vi "configure_new_target.vi"(11 "vsd":refnum<k24>) -> ()   [LabVIEW 2020]
uses:
  controls/target_configuration_cluster.ctl
  controls/thread_configuration_data.ctl
  controls/tx_transfer_group_configuration_data.ctl
  <vilib>/addons/VeriStand Custom Device Scripting APIs/Data Sharing Framework/DSF Core.lvlibp/Typedefs/DSF Timing Info.ctl
  controls/tx_configuration_data.ctl
  controls/rx_transfer_group_configuration_data.ctl
  controls/rx_configuration_data.ctl
  NationalInstruments.VeriStand.SystemDefinitionAPI
  <vilib>/addons/VeriStand Custom Device Scripting APIs/Data Sharing Framework/DSF Core.lvlibp
panel:
  in  "Remove RX Transfer Group":bool
  in  "Remove RX Connection":bool
  in  "Clear Configuration":bool
  in  "Remove Thread":bool
  in  "Remove TX Transfer Group":bool
  in  "Remove TX Connection":bool
  in  "Finish":bool
  in  "Cancel":bool
  in  "Target Plugin Timing":T1={"priority"=10000, "decimation"=0, "offset"=0}
  in  "Target DSF Threads":T2[](array[typedef])
  in  "Target ID":T7={"Name"="", "IP"="", "Username"="", "Password"="", "Operating System"="Linux_x64"}
  # "Target Settings"
  # "DSF Configuration"
  # "* Decimation = 0 forces \nplugin to be inline with PCL"
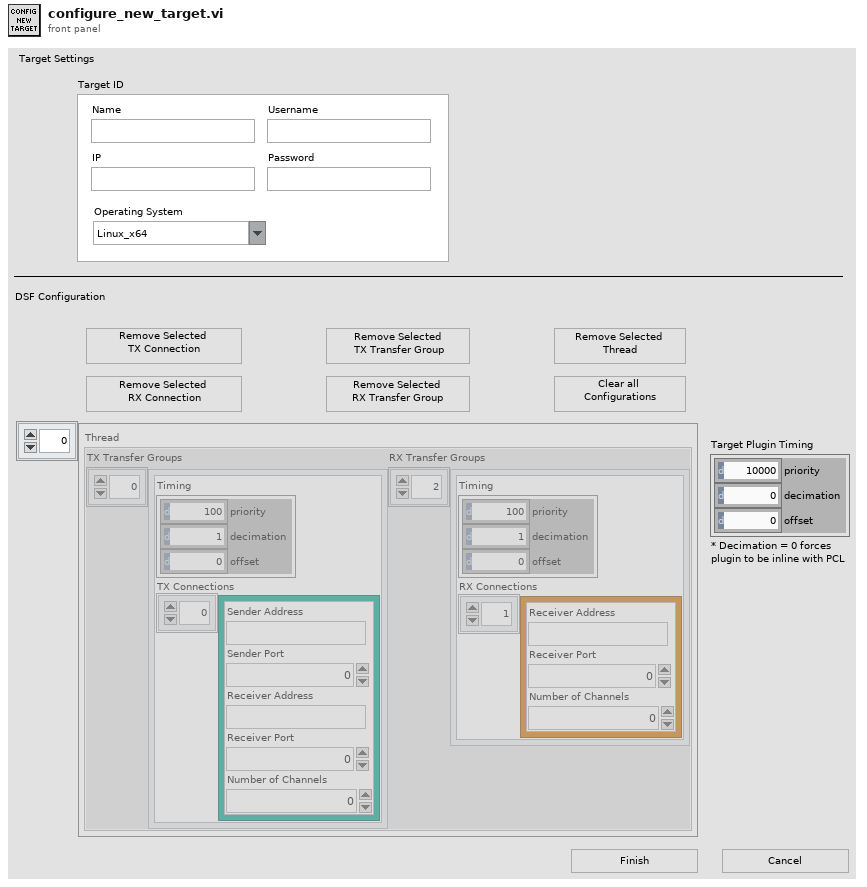
[diagram p1: front panel]
types:
  T1 = typedef "DSF Core.lvlibp/DSF Timing Info.ctl" = cluster{"priority":u64, "decimation":u64, "offset":u64}
  T2 = typedef "thread_configuration_data.ctl" = cluster{"TX Transfer Groups":T3[], "RX Transfer Groups":T5[]}
  T3 = typedef "tx_transfer_group_configuration_data.ctl" = cluster{"Timing":T1, "TX Connections":T4[]}
  T4 = typedef "tx_configuration_data.ctl" = cluster{"Sender Address":string, "Sender Port":u16, "Receiver Address":string, "Receiver Port":u16, "Number of Channels":u16}
  T5 = typedef "rx_transfer_group_configuration_data.ctl" = cluster{"Timing":T1, "RX Connections":T6[]}
  T6 = typedef "rx_configuration_data.ctl" = cluster{"Receiver Address":string, "Receiver Port":u16, "Number of Channels":u16}
  T7 = typedef "target_configuration_cluster.ctl" = cluster{"Name":string, "IP":string, "Username":string, "Password":string, "Operating System":string}
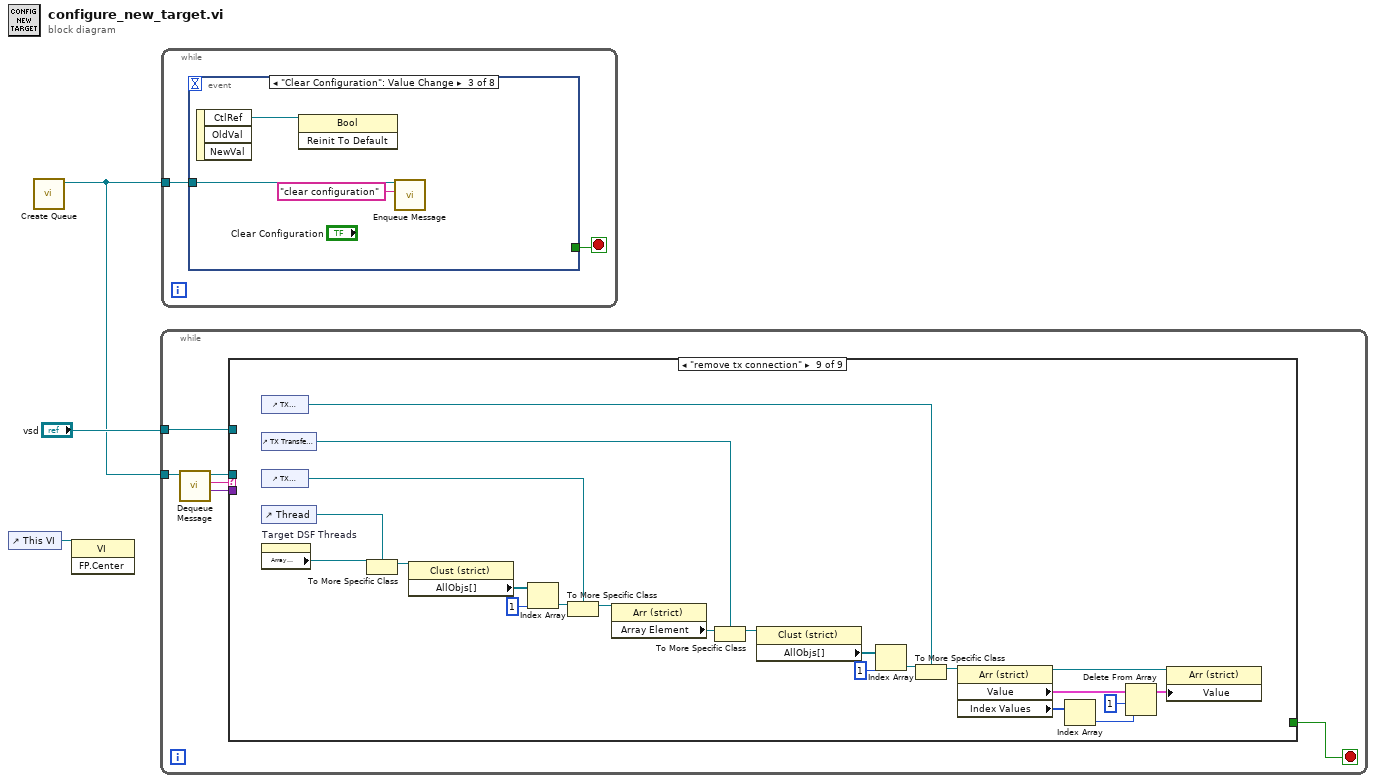
[diagram p0: block diagram]
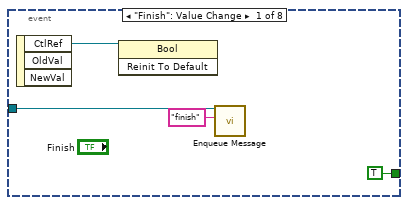
[diagram p2: hidden frame]
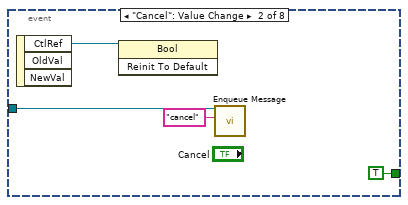
[diagram p3: hidden frame]
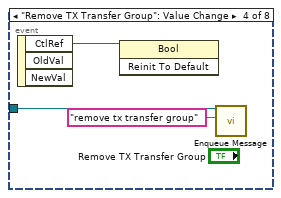
[diagram p4: hidden frame]
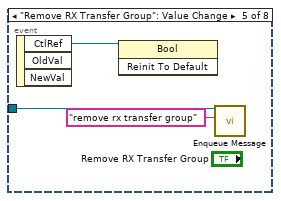
[diagram p5: hidden frame]
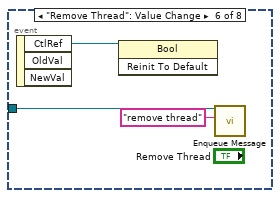
[diagram p6: hidden frame]
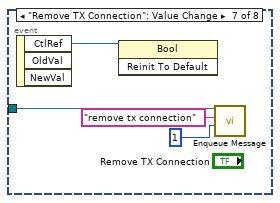
[diagram p7: hidden frame]
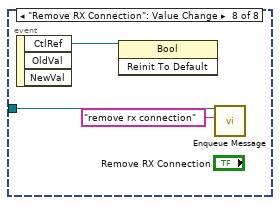
[diagram p8: hidden frame]
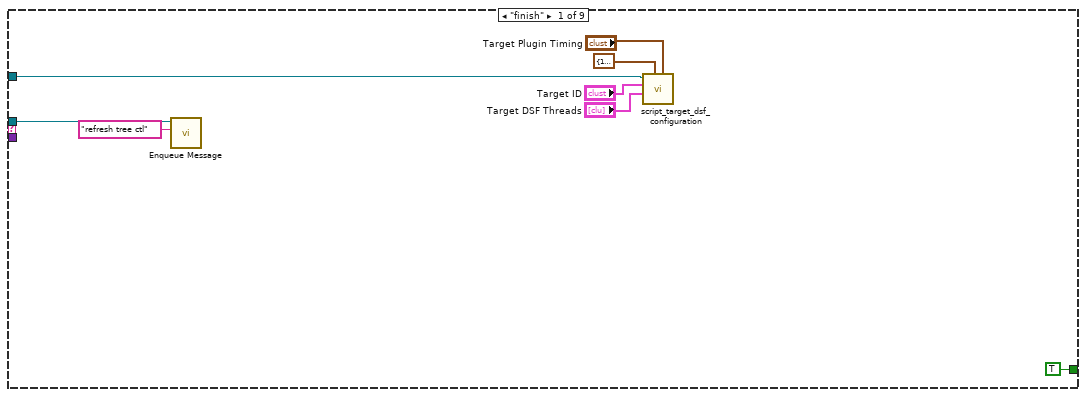
[diagram p9: hidden frame]
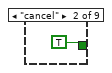
[diagram p10: hidden frame]
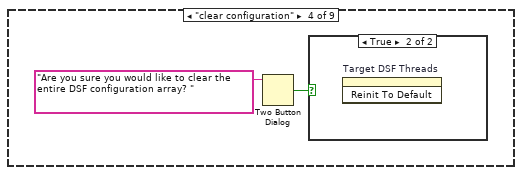
[diagram p12: hidden frame]
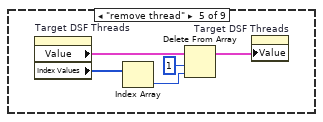
[diagram p14: hidden frame]
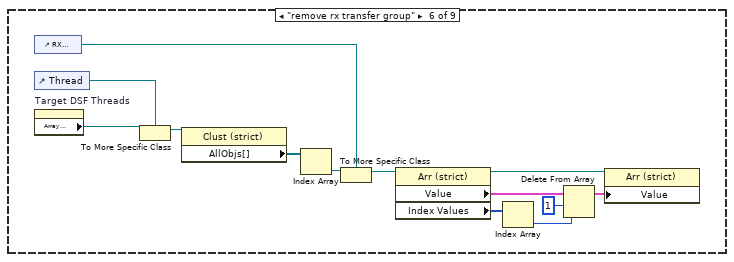
[diagram p15: hidden frame]
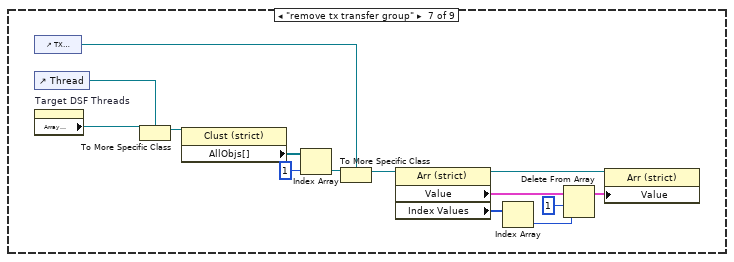
[diagram p16: hidden frame]
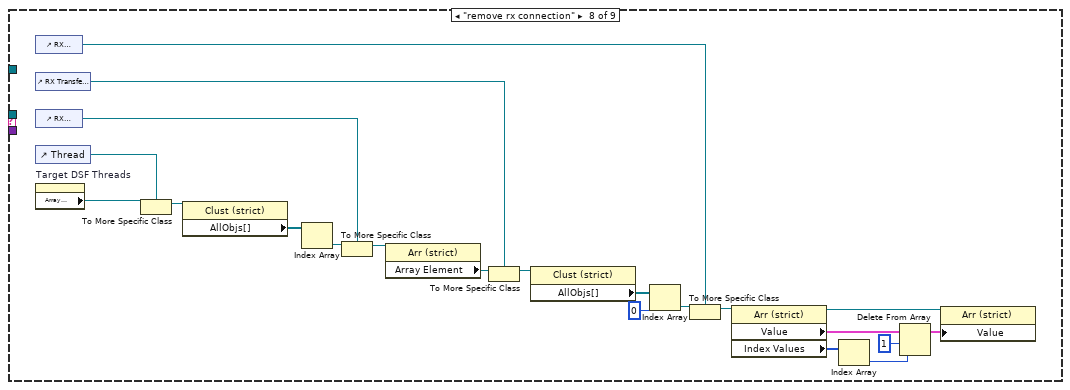
[diagram p17: hidden frame]
diagram:
  n1 = control-ref of="This VI"() -> (w1:refnum<vi>)
  n2 = call "Create Queue.vi"() -> ("Message Queue Out"=w2:refnum<queue>)  [unwired: 10 in, 1 out]
  n3 = invoke class="VI" method="FP.Center"(reference=w1) -> ()  [unwired: 2 in, 3 out]
  n4 = while {
    tunnel: w2 -> [w8]
    tunnel: "vsd" -> [w5]
    stop <- w4 stop-if-true
    n5 = call "Dequeue Message.vi"("Message Queue"=w8) -> ("Message Data"=w6:variant, "Message"=w9:string, "dup Message Queue"=w7:refnum<queue>)  [unwired: 7 in, 1 out]
    n6 = case shown="\"remove tx connection\"" w9 {
      tunnel: w7 -> [w16 _ _ _ _ _ _ _ _]
      tunnel: w6 -> [_ _ _ _ _ _ _ _ _]
      tunnel: w5 -> [w12 _ _ _ _ _ _ _ _]
      tunnel: [TRUE TRUE _ _ _ _ _ _ _] -> w4
      frame "finish" {
        n7 = call "Enqueue Message.vi"("Message"="refresh tree ctl", "Message Queue"=w16) -> ()  [unwired: 8 in, 2 out]
        n8 = call "script_target_dsf_configuration.vi"("Plugin Timing"="Target Plugin Timing", "configuration version"=cluster{"major":u32, "minor":u32, "fix":u32} {"major"=1, "minor"=0, "fix"=0}, "Target Threads"="Target DSF Threads", "Target Configuration"="Target ID", "vsd reference"=w12) -> ()  [unwired: 6 in, 1 out]
      }
      frame "cancel" {
      }
      frame Default {
      }
      frame "clear configuration" {
        n9 = Two Button Dialog(message="Are you sure you would like to clear the entire DSF configuration array? ") -> (T button?=w19:bool)  [unwired: 2 in]
        n10 = case shown="True" w19 {
          frame False {
          }
          frame True {
            n11 = invoke on="Target DSF Threads" class="Arr (strict)" method="Reinit To Default"() -> ()  [unwired: 3 in, 3 out]
          }
        }
      }
      frame "remove thread" {
        n12 = property on="Target DSF Threads" class="Arr (strict)"() -> ("Value"=w24:T2[], "Index Values"=w25:u32[])  [unwired: 2 in, 2 out]
        n13 = Index Array(array=w25) -> (element=w22:u32)  [unwired: 1 in]
        n14 = Delete From Array(array=w24, length=1, index=w22) -> (array with subset deleted=w21:T2[])  [unwired: 1 out]
        n15 = property on="Target DSF Threads" class="Arr (strict)"("Value"=w21) -> ()  [unwired: 2 in, 2 out]
      }
      frame "remove rx transfer group" {
        n16 = control-ref of="RX Transfer Groups"() -> (w27:refnum<vi>)
        n17 = control-ref of="Thread"() -> (w34:refnum<vi>)
        n18 = property on="Target DSF Threads" class="Arr (strict)"() -> ("Array Element"=w38:refnum<vi>)  [unwired: 2 in, 2 out]
        n19 = To More Specific Class(target class=w34, reference=w38) -> (specific class reference=w37:refnum<vi>)  [unwired: 1 in, 1 out]
        n20 = property class="Clust (strict)"(reference=w37) -> ("AllObjs[]"=w36:refnum<vi>[])  [unwired: 1 in, 2 out]
        n21 = Index Array(array=w36) -> (element=w35:refnum<vi>)  [unwired: 1 in]
        n22 = To More Specific Class(target class=w27, reference=w35) -> (specific class reference=w26:refnum<vi>)  [unwired: 1 in, 1 out]
        n23 = property class="Arr (strict)"(reference=w26) -> (reference out=w33:refnum<vi>, "Value"=w29:T5[], "Index Values"=w31:u32[])  [unwired: 1 in, 1 out]
        n24 = Index Array(array=w31) -> (element=w30:u32)  [unwired: 1 in]
        n25 = Delete From Array(array=w29, length=1, index=w30) -> (array with subset deleted=w28:T5[])  [unwired: 1 out]
        n26 = property class="Arr (strict)"(reference=w33, "Value"=w28) -> ()  [unwired: 1 in, 2 out]
      }
      frame "remove tx transfer group" {
        n27 = control-ref of="TX Transfer Groups"() -> (w41:refnum<vi>)
        n28 = control-ref of="Thread"() -> (w48:refnum<vi>)
        n29 = property on="Target DSF Threads" class="Arr (strict)"() -> ("Array Element"=w52:refnum<vi>)  [unwired: 2 in, 2 out]
        n30 = To More Specific Class(target class=w48, reference=w52) -> (specific class reference=w51:refnum<vi>)  [unwired: 1 in, 1 out]
        n31 = property class="Clust (strict)"(reference=w51) -> ("AllObjs[]"=w50:refnum<vi>[])  [unwired: 1 in, 2 out]
        n32 = Index Array(array=w50, index=1) -> (element=w49:refnum<vi>)
        n33 = To More Specific Class(target class=w41, reference=w49) -> (specific class reference=w40:refnum<vi>)  [unwired: 1 in, 1 out]
        n34 = property class="Arr (strict)"(reference=w40) -> (reference out=w47:refnum<vi>, "Value"=w43:T3[], "Index Values"=w45:u32[])  [unwired: 1 in, 1 out]
        n35 = Index Array(array=w45) -> (element=w44:u32)  [unwired: 1 in]
        n36 = Delete From Array(array=w43, length=1, index=w44) -> (array with subset deleted=w42:T3[])  [unwired: 1 out]
        n37 = property class="Arr (strict)"(reference=w47, "Value"=w42) -> ()  [unwired: 1 in, 2 out]
      }
      frame "remove rx connection" {
        n38 = control-ref of="RX Connections"() -> (w64:refnum<vi>)
        n39 = control-ref of="RX Transfer Group"() -> (w68:refnum<vi>)
        n40 = control-ref of="RX Transfer Groups"() -> (w56:refnum<vi>)
        n41 = control-ref of="Thread"() -> (w69:refnum<vi>)
        n42 = property on="Target DSF Threads" class="Arr (strict)"() -> ("Array Element"=w73:refnum<vi>)  [unwired: 2 in, 2 out]
        n43 = To More Specific Class(target class=w69, reference=w73) -> (specific class reference=w72:refnum<vi>)  [unwired: 1 in, 1 out]
        n44 = property class="Clust (strict)"(reference=w72) -> ("AllObjs[]"=w71:refnum<vi>[])  [unwired: 1 in, 2 out]
        n45 = Index Array(array=w71) -> (element=w70:refnum<vi>)  [unwired: 1 in]
        n46 = To More Specific Class(target class=w56, reference=w70) -> (specific class reference=w55:refnum<vi>)  [unwired: 1 in, 1 out]
        n47 = property class="Arr (strict)"(reference=w55) -> ("Array Element"=w54:refnum<vi>)  [unwired: 1 in, 2 out]
        n48 = To More Specific Class(target class=w68, reference=w54) -> (specific class reference=w67:refnum<vi>)  [unwired: 1 in, 1 out]
        n49 = property class="Clust (strict)"(reference=w67) -> ("AllObjs[]"=w65:refnum<vi>[])  [unwired: 1 in, 2 out]
        n50 = Index Array(array=w65, index=0) -> (element=w66:refnum<vi>)
        n51 = To More Specific Class(target class=w64, reference=w66) -> (specific class reference=w61:refnum<vi>)  [unwired: 1 in, 1 out]
        n52 = property class="Arr (strict)"(reference=w61) -> (reference out=w63:refnum<vi>, "Value"=w58:T6[], "Index Values"=w60:u32[])  [unwired: 1 in, 1 out]
        n53 = Index Array(array=w60) -> (element=w59:u32)  [unwired: 1 in]
        n54 = Delete From Array(array=w58, length=1, index=w59) -> (array with subset deleted=w57:T6[])  [unwired: 1 out]
        n55 = property class="Arr (strict)"(reference=w63, "Value"=w57) -> ()  [unwired: 1 in, 2 out]
      }
      frame "remove tx connection" {
        n56 = control-ref of="TX Connections"() -> (w86:refnum<vi>)
        n57 = control-ref of="TX Transfer Group"() -> (w90:refnum<vi>)
        n58 = control-ref of="TX Transfer Groups"() -> (w78:refnum<vi>)
        n59 = control-ref of="Thread"() -> (w91:refnum<vi>)
        n60 = property on="Target DSF Threads" class="Arr (strict)"() -> ("Array Element"=w95:refnum<vi>)  [unwired: 2 in, 2 out]
        n61 = To More Specific Class(target class=w91, reference=w95) -> (specific class reference=w94:refnum<vi>)  [unwired: 1 in, 1 out]
        n62 = property class="Clust (strict)"(reference=w94) -> ("AllObjs[]"=w93:refnum<vi>[])  [unwired: 1 in, 2 out]
        n63 = Index Array(array=w93, index=1) -> (element=w92:refnum<vi>)
        n64 = To More Specific Class(target class=w78, reference=w92) -> (specific class reference=w77:refnum<vi>)  [unwired: 1 in, 1 out]
        n65 = property class="Arr (strict)"(reference=w77) -> ("Array Element"=w76:refnum<vi>)  [unwired: 1 in, 2 out]
        n66 = To More Specific Class(target class=w90, reference=w76) -> (specific class reference=w89:refnum<vi>)  [unwired: 1 in, 1 out]
        n67 = property class="Clust (strict)"(reference=w89) -> ("AllObjs[]"=w87:refnum<vi>[])  [unwired: 1 in, 2 out]
        n68 = Index Array(array=w87, index=1) -> (element=w88:refnum<vi>)
        n69 = To More Specific Class(target class=w86, reference=w88) -> (specific class reference=w83:refnum<vi>)  [unwired: 1 in, 1 out]
        n70 = property class="Arr (strict)"(reference=w83) -> (reference out=w85:refnum<vi>, "Value"=w80:T4[], "Index Values"=w82:u32[])  [unwired: 1 in, 1 out]
        n71 = Index Array(array=w82) -> (element=w81:u32)  [unwired: 1 in]
        n72 = Delete From Array(array=w80, length=1, index=w81) -> (array with subset deleted=w79:T4[])  [unwired: 1 out]
        n73 = property class="Arr (strict)"(reference=w85, "Value"=w79) -> ()  [unwired: 1 in, 2 out]
      }
    }
  }
  n74 = while {
    tunnel: w2 -> [w97]
    stop <- w96 stop-if-true
    n75 = event shown="[2] \"Clear Configuration\": Value Change" {
      selector: _ -> [_ _ _ _ _ _ _ _]
      dyn-events: _ -> [_ _ _ _ _ _ _ _]
      timeout: _ -> [_ _ _ _ _ _ _ _]
      tunnel: w97 -> [w101 w105 w108 w111 w114 w117 w121 w124]
      tunnel: [TRUE TRUE _ _ _ _ _ _] -> w96
      event "Finish": Value Change {
        n76 = event-data() -> ("CtlRef"=w99:refnum<vi>)  [unwired: 1 in, 2 out]
        n77 = invoke class="Bool" method="Reinit To Default"(reference=w99) -> ()  [unwired: 2 in, 3 out]
        n78 = call "Enqueue Message.vi"("Message"="finish", "Message Queue"=w101) -> ()  [unwired: 8 in, 2 out]
      }
      event "Cancel": Value Change {
        n79 = event-data() -> ("CtlRef"=w103:refnum<vi>)  [unwired: 1 in, 2 out]
        n80 = invoke class="Bool" method="Reinit To Default"(reference=w103) -> ()  [unwired: 2 in, 3 out]
        n81 = call "Enqueue Message.vi"("Message"="cancel", "Message Queue"=w105) -> ()  [unwired: 8 in, 2 out]
      }
      event "Clear Configuration": Value Change {
        n82 = event-data() -> ("CtlRef"=w106:refnum<vi>)  [unwired: 1 in, 2 out]
        n83 = invoke class="Bool" method="Reinit To Default"(reference=w106) -> ()  [unwired: 2 in, 3 out]
        n84 = call "Enqueue Message.vi"("Message"="clear configuration", "Message Queue"=w108) -> ()  [unwired: 8 in, 2 out]
      }
      event "Remove TX Transfer Group": Value Change {
        n85 = event-data() -> ("CtlRef"=w109:refnum<vi>)  [unwired: 1 in, 2 out]
        n86 = invoke class="Bool" method="Reinit To Default"(reference=w109) -> ()  [unwired: 2 in, 3 out]
        n87 = call "Enqueue Message.vi"("Message"="remove tx transfer group", "Message Queue"=w111) -> ()  [unwired: 8 in, 2 out]
      }
      event "Remove RX Transfer Group": Value Change {
        n88 = event-data() -> ("CtlRef"=w112:refnum<vi>)  [unwired: 1 in, 2 out]
        n89 = invoke class="Bool" method="Reinit To Default"(reference=w112) -> ()  [unwired: 2 in, 3 out]
        n90 = call "Enqueue Message.vi"("Message"="remove rx transfer group", "Message Queue"=w114) -> ()  [unwired: 8 in, 2 out]
      }
      event "Remove Thread": Value Change {
        n91 = event-data() -> ("CtlRef"=w115:refnum<vi>)  [unwired: 1 in, 2 out]
        n92 = invoke class="Bool" method="Reinit To Default"(reference=w115) -> ()  [unwired: 2 in, 3 out]
        n93 = call "Enqueue Message.vi"("Message"="remove thread", "Message Queue"=w117) -> ()  [unwired: 8 in, 2 out]
      }
      event "Remove TX Connection": Value Change {
        n94 = event-data() -> ("CtlRef"=w119:refnum<vi>)  [unwired: 1 in, 2 out]
        n95 = invoke class="Bool" method="Reinit To Default"(reference=w119) -> ()  [unwired: 2 in, 3 out]
        n96 = call "Enqueue Message.vi"("Data"=1 ("index"), "Message"="remove tx connection", "Message Queue"=w121) -> ()  [unwired: 7 in, 2 out]
      }
      event "Remove RX Connection": Value Change {
        n97 = event-data() -> ("CtlRef"=w122:refnum<vi>)  [unwired: 1 in, 2 out]
        n98 = invoke class="Bool" method="Reinit To Default"(reference=w122) -> ()  [unwired: 2 in, 3 out]
        n99 = call "Enqueue Message.vi"("Message"="remove rx connection", "Message Queue"=w124) -> ()  [unwired: 8 in, 2 out]
      }
    }
  }
